vi "11- Peak detector.vi"() -> ()   [LabVIEW 2019]
panel:
  in  "Input Peak level":dbl=10.0 format="%#_13g"
  out "Number of Peaks":i32
  out "Indexes of the Peaks":dbl[](array[numeric])
  out "Array":dbl[](array[numeric])
  # "PEAK DETECTOR"
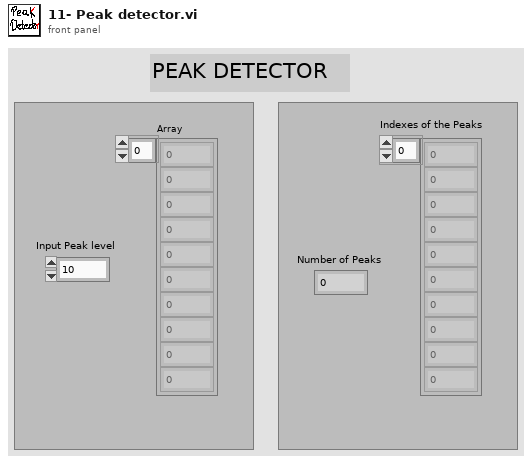
[diagram p1: front panel]
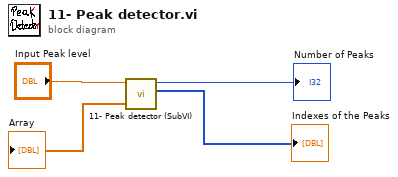
[diagram p0: block diagram]
diagram:
  n1 = call "11- Peak detector (SubVI).vi"("Input peak level"="Input Peak level") -> ("Number of peaks"=→"Number of Peaks":i32, "Indexes of peaks"=→"Indexes of the Peaks":i32[], "Array"=→"Array":dbl[])  [unwired: 8 in]
